vi "Zaber T read current position.vi"(8 "error in (no error)":errorcluster, 10 "Device Number (LV)":u8, 11 "VISA Refnum in":refnum<visa-resource-name>) -> (0 "error out":errorcluster, 2 "Current position (LV)":i32, 3 "VISA Refnum out":refnum<visa-resource-name>)   [LabVIEW 2013]
uses:
  <instrlib>/ZaberTSeries/Public/Utility/Response.ctl
  <instrlib>/ZaberTSeries/ZaberTSeries.lvlib
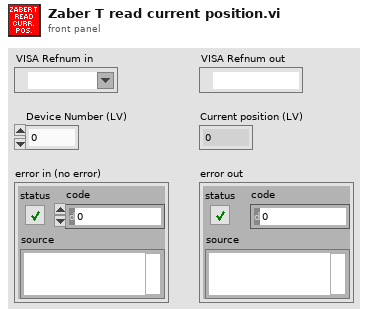
[diagram p1: front panel]
types:
  T1 = typedef "ZaberTSeries.lvlib/Response.ctl" = cluster{"Device Number":u8, "Command":u8, "Data":i32}
  T2 = cluster{"Device Number (LV)":u8, "Command":u8, "Data":i32, "Response Count":i32}
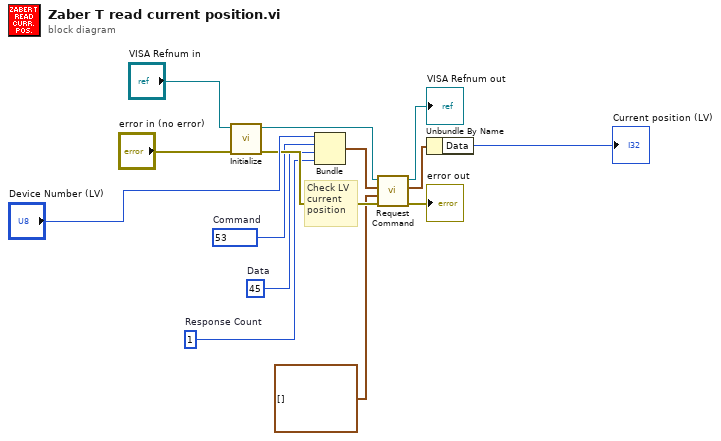
[diagram p0: block diagram]
diagram:
  w3 = 45  # Data
  w5 = 1  # Response Count
  w2 = u8 53 items=["Echo"=55, "Home"=1, "Move Absolute"=20, "Move Relative"=21, "Move at Constant Speed"=22, "Renumber"=2, "Restore Settings"=36, "Stop"=23]  # Command
  # "Check LV\ncurrent \nposition"
  n1 = call <instrlib>:"Initialize.vi"("error in (no error)"="error in (no error)", "VISA resource name"="VISA Refnum in") -> ("error out"=w10:errorcluster, "VISA resource name out"=w8:refnum<visa-resource-name>)  [unwired: 7 in, 1 out]
  n2 = Bundle("Device Number (LV)"="Device Number (LV)", "Command"=w2, "Data"=w3, "Response Count"=w5) -> (w4:T2)  [unwired: 1 in]
  n3 = call <instrlib>:"Request Command.vi"("error in (no error)"=w10, "Responses in"=T1[] [], "Request"=w4, "VISA resource name"=w8) -> ("error out"=→"error out":errorcluster, "First Response"=w7:T1, "VISA resource name out"=→"VISA Refnum out":refnum<visa-resource-name>)  [unwired: 4 in, 1 out]
  n4 = Unbundle By Name(w7) -> ("Data"=→"Current position (LV)":i32)
